vi "TSM SSC Digital Write Source Waveform [Broadcast].vi"(0 "Digital TSM In":T1, 1 "Waveform Name":string, 5 "Waveform Data":u32[](array[numeric]) format="%.0x", 7 "Expand to Minimum Size?":bool caption="Expand to Minimum Size? (F)", 9 "Minimum Size":i32=128 caption="Minimum Size (128)", 11 "error in":errorcluster) -> (4 "Digital TSM Out":T1, 15 "error out":errorcluster)   [LabVIEW 2019]
doc: "Writes the same waveform data to all sites connected to the specified pin(s) and pin group(s). Use this instance of the niDigital Write Source Waveform VI if you set the data mapping parameter of your source waveform to Broadcast."
uses:
  TSM/TSM SSC Digital.ctl
  <vilib>/NI_TestStand_SemiconductorModule/NI_TestStand_Semiconductor_Module.lvlibp/PinMap/Digital Pattern/PinQueryContext/DigitalPatternPinQueryContext.lvclass
  SSC Digital/SSC Digital.ctl
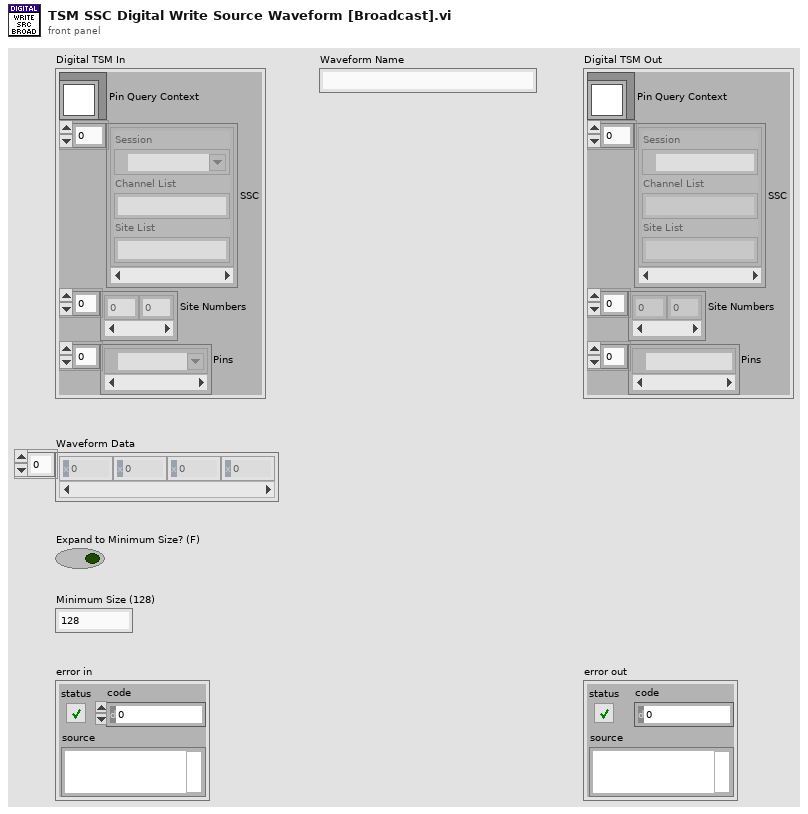
[diagram p1: front panel]
types:
  T1 = typedef "TSM SSC Digital.ctl" = cluster{"Pin Query Context":refnum<class "DigitalPatternPinQueryContext.lvclass">, "SSC":T2[], "Site Numbers":i32[], "Pins":tag[]}
  T2 = typedef "SSC Digital.ctl" = cluster{"Session":refnum<k15>, "Channel List":string, "Site List":string}
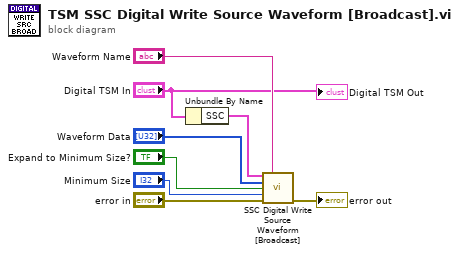
[diagram p0: block diagram]
diagram:
  n1 = Unbundle By Name("Digital TSM In") -> ("SSC"=w2:T2[])
  n2 = call "SSC Digital Write Source Waveform [Broadcast].vi"("Digital SSC in"=w2, "Waveform Name"="Waveform Name", "Waveform Data"="Waveform Data", "Expand to Minimum Size?"="Expand to Minimum Size?", "Minimum Size"="Minimum Size", "error in"="error in") -> ("error out"=→"error out":errorcluster)  [unwired: 8 in, 1 out]
  "Digital TSM Out" <- "Digital TSM In"
